vi "Turn To Angle.vi"(11 "Angle":dbl) -> ()   [LabVIEW 2015]
uses:
  <vilib>/Rock Robotics/WPI/Framework/Command Status Info.ctl
  <vilib>/Rock Robotics/WPI/Framework/Completion Status.ctl
  <vilib>/Rock Robotics/WPI/Framework/Completion Notifier.ctl
  Implementation/Angular PID Setpoints.ctl
  Implementation/Angular PID Operations.ctl
panel:
  out "SubSystem Data":T1
  out "Command Info":T3
  in  "Command Info 2":T3
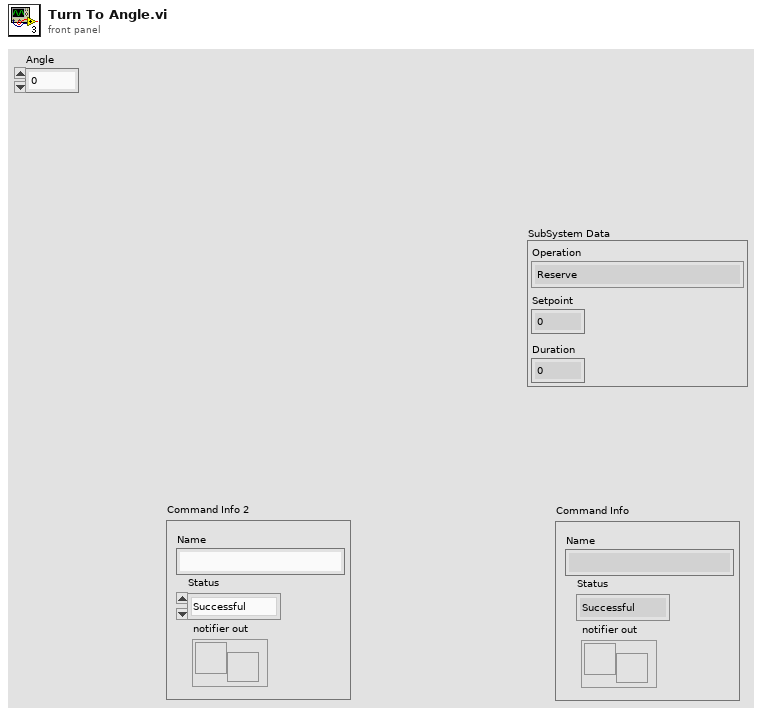
[diagram p1: front panel]
types:
  T1 = typedef "Angular PID Setpoints.ctl" = cluster{"Operation":T2, "Setpoint":dbl, "Duration":dbl}
  T2 = typedef "Angular PID Operations.ctl" = enum16{"Reserve", "Read Current", "Immediate", "Turn To Angle"}
  T3 = typedef "Command Status Info.ctl" = cluster{"Name":string, "Status":T4, "notifier out":T5}
  T4 = typedef "Completion Status.ctl" = enum16{"Successful", "Aborted", "Incomplete"}
  T5 = typedef "Completion Notifier.ctl" = refnum<notifier>
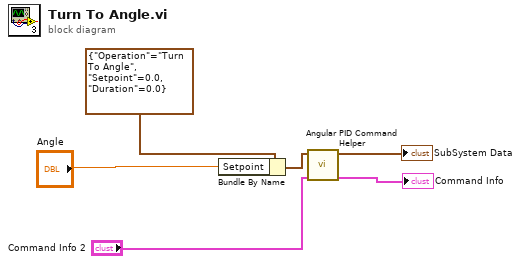
[diagram p0: block diagram]
diagram:
  n1 = Bundle By Name(cluster=T1 {"Operation"=enum."Turn To Angle", "Setpoint"=0.0, "Duration"=0.0} ("SubSystem Data"), "Setpoint"="Angle") -> (w2:T1)
  n2 = call "Angular PID Command Helper.vi"("Command Info In"="Command Info 2", "SubSystem Data"=w2) -> ("Command Info Out"=→"Command Info":T3, "SubSystem Data"=→"SubSystem Data":T1)  [unwired: 8 in]
